vi "Run VI Without Panel.vi"(8 "error in":errorcluster, 11 "VI Name":string) -> (0 "error out":errorcluster, 3 "vi reference":refnum<vi>)   [LabVIEW 2018]
doc: "啟動VI，並使其在背景執行"
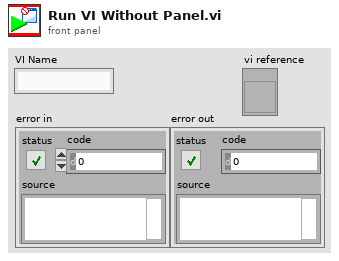
[diagram p1: front panel]
types:
  T1 = enum32{"Bad", "Idle", "Run top level", "Running"}
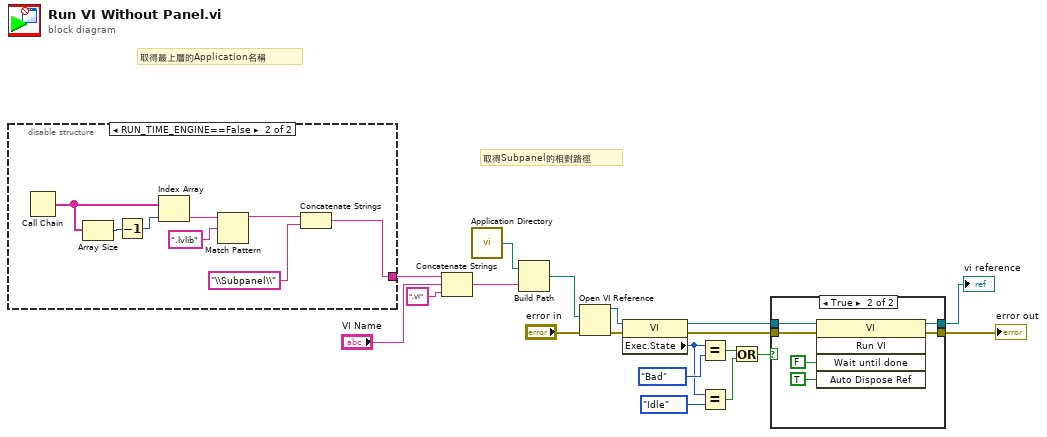
[diagram p0: block diagram]
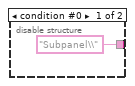
[diagram p2: hidden frame]
diagram:
  # "取得Subpanel的相對路徑"
  # "取得最上層的Application名稱"
  n1 = disable-structure shown="RUN_TIME_ENGINE==False" {
    disable-tunnel: ["Subpanel\\" ("name or relative path") w24] -> w1
    frame condition #0 {
    }
    frame condition #1 (active) {
      n2 = Call Chain() -> (call chain=w23:string[])
      n3 = Array Size(array=w23) -> (size(s)=w22:i32)
      n4 = Decrement(x=w22) -> (x-1=w21:i32)
      n5 = Index Array(array=w23, index=w21) -> (element=w27:string)
      n6 = Match Pattern(string=w27, regular expression=".lvlib") -> (before substring=w26:string)  [unwired: 1 in, 3 out]
      n7 = Concatenate Strings(w26, "\\Subpanel\\" ("name or relative path")) -> (w24:string)
    }
  }
  n8 = Concatenate Strings(w1, "VI Name", ".vi" ("string")) -> (w8:string)
  n9 = call <vilib>:"Application Directory.vi"() -> ("Application Directory"=w9:path)
  n10 = Build Path(base path=w9, name or relative path=w8) -> (appended path=w5:path)
  n11 = Open VI Reference(vi path=w5, error in (no error)="error in") -> (vi reference=w3:refnum<vi>, error out=w2:errorcluster)  [unwired: 4 in]
  n12 = property class="VI"(reference=w3, error in=w2) -> (reference out=w16:refnum<vi>, error out=w15:errorcluster, "Exec.State"=w10:T1)
  n13 = Equal?(x=w10, y=T1."Bad" ("Execution:State")) -> (x = y?=w17:bool)
  n14 = Equal?(x=w10, y=T1."Idle" ("Execution:State")) -> (x = y?=w11:bool)
  n15 = Or(x=w17, y=w11) -> (x .or. y?=w12:bool)
  n16 = case shown="True" w12 {
    tunnel: w16 -> [w29 w33]
    tunnel: w15 -> [w30 w32]
    tunnel: [w30 w35] -> w14
    tunnel: [w29 w31] -> w13
    frame False {
    }
    frame True {
      n17 = invoke class="VI" method="Run VI"(reference=w33, error in=w32, "Wait until done"=FALSE ("Wait Until Done"), "Auto Dispose Ref"=TRUE ("Auto Dispose Reference")) -> (reference out=w31:refnum<vi>, error out=w35:errorcluster)  [unwired: 1 in, 3 out]
    }
  }
  "error out" <- w14
  "vi reference" <- w13
